vi "判断.vi"(0 "y 3":dbl=65.0 format="%#_13g", 4 "y2-2":dbl, 6 "y2-1":dbl=70.0 format="%#_13g", 8 "y":dbl, 9 "x 3":dbl, 10 "x 2":dbl, 11 "x":dbl) -> (1 "非x? 3":bool, 2 "非x? 2":bool, 3 "非x?":bool)   [LabVIEW 2013]
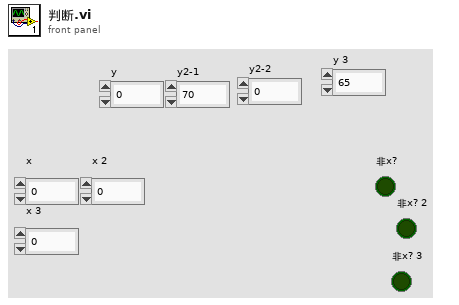
[diagram p1: front panel]
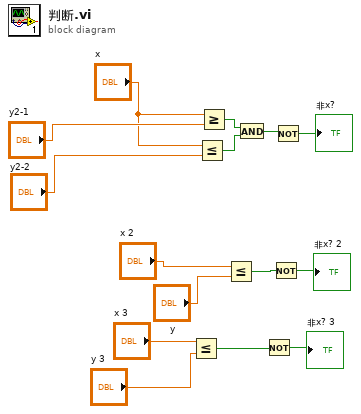
[diagram p0: block diagram]
diagram:
  n1 = Less Or Equal?(x="x 3", y="y 3") -> (x <= y?=w13:bool)
  n2 = Less Or Equal?(x="x", y="y2-2") -> (x <= y?=w14:bool)
  n3 = Greater Or Equal?(x="x", y="y2-1") -> (x >= y?=w15:bool)
  n4 = Less Or Equal?(x="x 2", y="y") -> (x <= y?=w7:bool)
  n5 = And(x=w15, y=w14) -> (x .and. y?=w1:bool)
  n6 = Not(x=w13) -> (.not. x?=→"非x? 3":bool)
  n7 = Not(x=w7) -> (.not. x?=→"非x? 2":bool)
  n8 = Not(x=w1) -> (.not. x?=→"非x?":bool)
